vi "(SubVI) Theme combination data.vi"() -> (1 "Talent order CB":string[](array[string]), 2 "arr Description CB":string[](array[string]))   [LabVIEW 2024]
panel:
  out "min Talent 2":string
  out "min Talent 1":string
  out "max Talent 1":string
  out "max Talent 2":string
  out "min description":string
  out "max description":string
  out "min string length":i32
  out "max string length":i32
  out "string":string
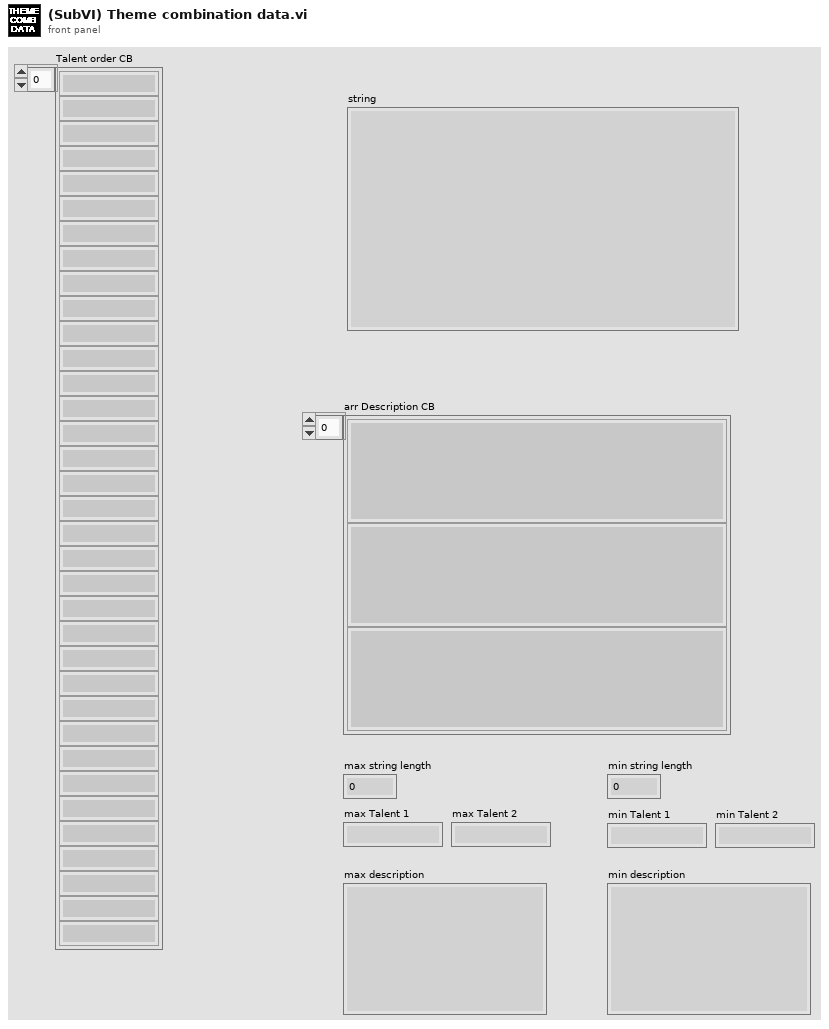
[diagram p1: front panel]
types:
  T1 = enum16{"open", "replace", "create", "open or create", "replace or create", "replace or create with confirmation"}
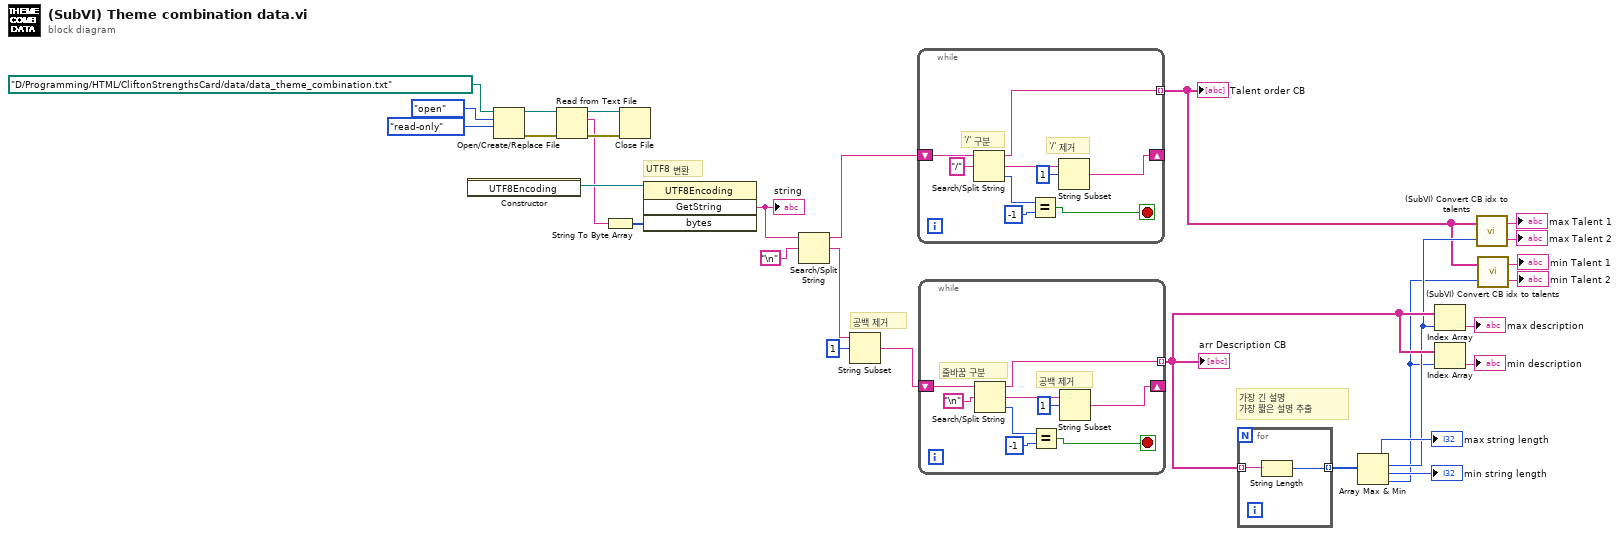
[diagram p0: block diagram]
diagram:
  # "가장 긴 설명\n가장 짧은 설명 추출"
  # "공백 제거"
  # "UTF8 변환"
  n1 = constructor class="UTF8Encoding"() -> (reference out=w22:refnum<k24>)  [unwired: 3 in, 2 out]
  n2 = Open/Create/Replace File(file path (use dialog)=path "D:/Programming/HTML/CliftonStrengthsCard/data/data_theme_combination.txt" ("Path 3"), operation (0:open)=T1."open", access (0:read/write)=enum16{"read/write", "read-only", "write-only"}."read-only") -> (refnum out=w29:refnum<file>, error out=w27:errorcluster)  [unwired: 3 in, 1 out]
  n3 = Read from Text File(file (use dialog)=w29, error in=w27) -> (refnum out=w28:refnum<file>, text=w21:string, error out=w26:errorcluster)  [unwired: 2 in, 1 out]
  n4 = String To Byte Array(string=w21) -> (unsigned byte array=w20:u8[])
  n5 = Close File(refnum=w28, error in=w26) -> ()  [unwired: 2 out]
  n6 = invoke class="UTF8Encoding" method="GetString"(reference=w22, "bytes"=w20) -> ("GetString"=w19:string)  [unwired: 2 in, 3 out]
  "string" <- w19
  n7 = Search/Split String(string=w19, search string/char (-)="\n") -> (substring before match=w15:string, match + rest of string=w17:string)  [unwired: 1 in, 1 out]
  n8 = String Subset(string=w17, offset (0)=1) -> (substring=w14:string)  [unwired: 1 in]
  n9 = while {
    shift-right: [w33] -> _
    shift-left: w15 -> [w38]
    tunnel: [w36] -> w2 mode=indexing
    stop <- w31 stop-if-true
    # "'/' 구분"
    # "'/' 제거"
    n10 = Search/Split String(string=w38, search string/char (-)="/") -> (substring before match=w36:string, match + rest of string=w34:string, offset of match=w32:i32)  [unwired: 1 in]
    n11 = Equal?(x=w32, y=-1 ("offset (0)")) -> (x = y?=w31:bool)
    n12 = String Subset(string=w34, offset (0)=1) -> (substring=w33:string)  [unwired: 1 in]
  }
  "Talent order CB" <- w2
  n13 = while {
    shift-right: [w43] -> _
    shift-left: w14 -> [w47]
    tunnel: [w46] -> w8 mode=indexing
    stop <- w41 stop-if-true
    # "줄바꿈 구분"
    # "공백 제거"
    n14 = Search/Split String(string=w47, search string/char (-)="\n") -> (substring before match=w46:string, match + rest of string=w44:string, offset of match=w42:i32)  [unwired: 1 in]
    n15 = Equal?(x=w42, y=-1 ("offset (0)")) -> (x = y?=w41:bool)
    n16 = String Subset(string=w44, offset (0)=1) -> (substring=w43:string)  [unwired: 1 in]
  }
  "arr Description CB" <- w8
  n17 = for {
    tunnel: w8 -> [w49] mode=indexing
    tunnel: [w48] -> w13 mode=indexing
    n18 = String Length(string=w49) -> (length=w48:i32)
  }
  n19 = Array Max & Min(array=w13) -> (max value=→"max string length":i32, max index (indices)=w7:i32, min value=→"min string length":i32, min index (indices)=w1:i32)
  n20 = Index Array(array=w8, index=w7) -> (element=→"max description":string)
  n21 = Index Array(array=w8, index=w1) -> (element=→"min description":string)
  n22 = call "(SubVI) Convert CB idx to talents.vi"("index"=w7, "Talent order CB"=w2) -> ("Talent 2"=→"max Talent 2":string, "Talent 1"=→"max Talent 1":string)
  n23 = call "(SubVI) Convert CB idx to talents.vi"("index"=w1, "Talent order CB"=w2) -> ("Talent 2"=→"min Talent 2":string, "Talent 1"=→"min Talent 1":string)
